vi "Facade.vi"(0 "Data In":T8, 2 "Display State In":T4={"Numeric"=0.0, "Timeline Ref"=refnum, "Waveform Ref"=refnum, "Fill Plots"=FALSE, "Cursor Redraw"=TRUE}, 3 "Container State":T7) -> (6 "Data Out":T8, 7 "Display State Out":T4={"Numeric"=0.0, "Timeline Ref"=refnum, "Waveform Ref"=refnum, "Fill Plots"=FALSE, "Cursor Redraw"=TRUE}, 8 "Action":T3)   [LabVIEW 2017, in "XGrapher.xctl"]
uses:
  XGrapher.xctl
  Data 1.ctl
  Typedefs/Xctrl-Data array.ctl
  Typedefs/Xcrtl-Data format definition.ctl
  Typedefs/Xctl-XY data type definition.ctl
  Typedefs/Xctrl-ROI type enum.ctl
  <vilib>/_xctls/Container State.ctl
  State 1.ctl
  Typedefs/Xctrl-Timeline graph ref.ctl
  Typedefs/Xctrl-Waveform graph ref.ctl
  <vilib>/_xctls/Action.ctl
  Typedefs/Xinformation.ctl
  Typedefs/Xcrtl-Click Operation.ctl
  <vilib>/Utility/miscctls.llb/LVPointTypeDef.ctl
  Globals/gl_X-Grapher refs.vi
  <vilib>/_xctls/XControlSupport.lvlib
panel:
  out "Points in graph":i32 format="%.0f points"
  out "Mouse coordinates info":string="Mouse: X=0, Y=0"
  out "Graph cursor coordinates info":string="Graph cursor: X=0, Y=0"
  out "Xinformation":T1
  out "XY Graph":T13(graph)
  out "Points in timeline":i32 format="%.0f points"
  out "Timeline Graph":T13(graph)
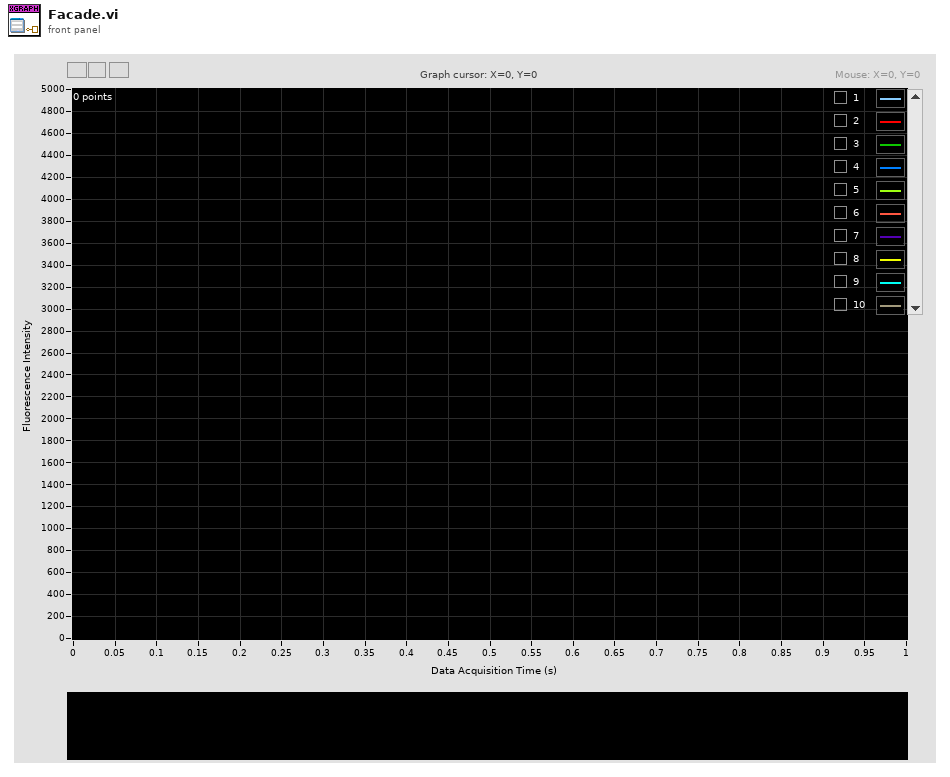
[diagram p1: front panel]
types:
  T1 = typedef "XGrapher.xctl/Xinformation.ctl" = cluster{"Cursor Span":dbl, "Icon":u16, "Mouse Down":bool, "Owning VI":refnum<vi>, "Mouse area":T2, "Dragging":bool, "Drag Offset":dbl, "Original Cursor Pos":cluster{"Left":dbl, "Right":dbl, "Span":dbl}, "Cursor Redraw":bool}
  T2 = typedef "XGrapher.xctl/Xcrtl-Click Operation.ctl" = enum16{"Move", "left cursor", "right cursor", "none"}
  T3 = typedef "XControlSupport.lvlib/Action.ctl" = cluster{"Data Changed?":bool, "State Changed?":bool, "Action Name":string}
  T4 = typedef "XGrapher.xctl/State 1.ctl" = cluster{"Numeric":dbl, "Timeline Ref":T5, "Waveform Ref":T6, "Fill Plots":bool, "Cursor Redraw":bool}
  T5 = typedef "XGrapher.xctl/Xctrl-Timeline graph ref.ctl" = refnum<vi>
  T6 = typedef "XGrapher.xctl/Xctrl-Waveform graph ref.ctl" = refnum<vi>
  T7 = typedef "XControlSupport.lvlib/Container State.ctl" = cluster{"Indicator?":bool, "Run Mode?":bool, " Refnum":refnum<vi>}
  T8 = typedef "XGrapher.xctl/Data 1.ctl" = cluster{"Data & info by ROI index":T9, "Index of selected plot":u16, "Points in each trial":i32, "POI Averaging":bool, "Reset graph X-axis scaling":bool, "Selected point index in MSCN (unity based)":u16}
  T9 = typedef "Xctrl-Data array.ctl" = T10[]
  T10 = typedef "XGrapher.xctl/Xcrtl-Data format definition.ctl" = cluster{"Plot.Plot Name":string, "Data":T11, "Timeline data":T11, "Type":T12, "Points per cycle":u16, "ROI index":u16}
  T11 = typedef "XGrapher.xctl/Xctl-XY data type definition.ctl" = cluster{"X-Axis values":sgl[], "Y-Axis values (s)":sgl[]}
  T12 = typedef "Xctrl-ROI type enum.ctl" = enum16{"POI", "Mini-scan", "Group"}
  T13 = cluster{"X-Axis values":sgl[], "Y-Axis values (s)":sgl[]}[]
  T14 = typedef "LVPointTypeDef.ctl" = cluster{"Horizontal":i16, "Vertical":i16}
  T15 = cluster{"XY Graph":refnum<vi>, "Timeline Graph":refnum<vi>}
  T16 = typedef "XGrapher.xctl/Xctrl-XY Graph data type definition.ctl" = T11[]
  T17 = typedef "LVPoint32TypeDef.ctl" = cluster{"Horizontal":i32, "Vertical":i32}
  T18 = typedef "LVRangeTypeDef.ctl" = cluster{"Minimum":dbl, "Maximum":dbl, "Increment":dbl, "Minor Increment":dbl, "Start":dbl}
  T19 = typedef "lveventtype.ctl" = enum32{"Null", "Timeout", "Annotation Menu Selection", "Annotation Menu Selection?", "App Instance Close", "App Instance Close?", "Autoscale Range Change", "Bookmark Info Change", "Cell Edit", "Cell Edit?", "Cursor Grab", "Cursor Grab?", "Cursor Menu Selection", "Cursor Menu Selection?", "Cursor Move", "Cursor Release", "Data Change", "Direction Change", "Display State Change", "Drag Ended", "Drag Enter", "Drag Leave", "Drag Over", "Drag Source Update", "Drag Starting", "Drag Starting?", "Drop", "Exec State Change", "Key Down", "Key Down?", "Key Repeat", "Key Repeat?", "Key Up", "Listbox Double Click", "Menu Activation?", "Menu Selection (App)", "Menu Selection? (App)", "Menu Selection (User)", "Mouse Down", "Mouse Down?", "Mouse Enter", "Mouse Leave", "Mouse Move", "Mouse Up", "Mouse Wheel", "NI Security User Change (App)", "Pane Size", "Panel Close", "Panel Close?", "Panel Resize", "Plot Attribute Change", "Scale Range Change", "Shortcut Menu Activation?", "Shortcut Menu Selection (App)", "Shortcut Menu Selection? (App)", "Shortcut Menu Selection (User)", "Tree Double Click", "Tree Drag", "Tree Drag?", "Tree Drop", "Tree Drop?", "Tree Item Close", "Tree Item Close?", "Tree Item Open", "Tree Item Open?", "User Event", "Value Change"}
  T20 = cluster{"Left cursor pos.":dbl, "Left cursor pos.":dbl}
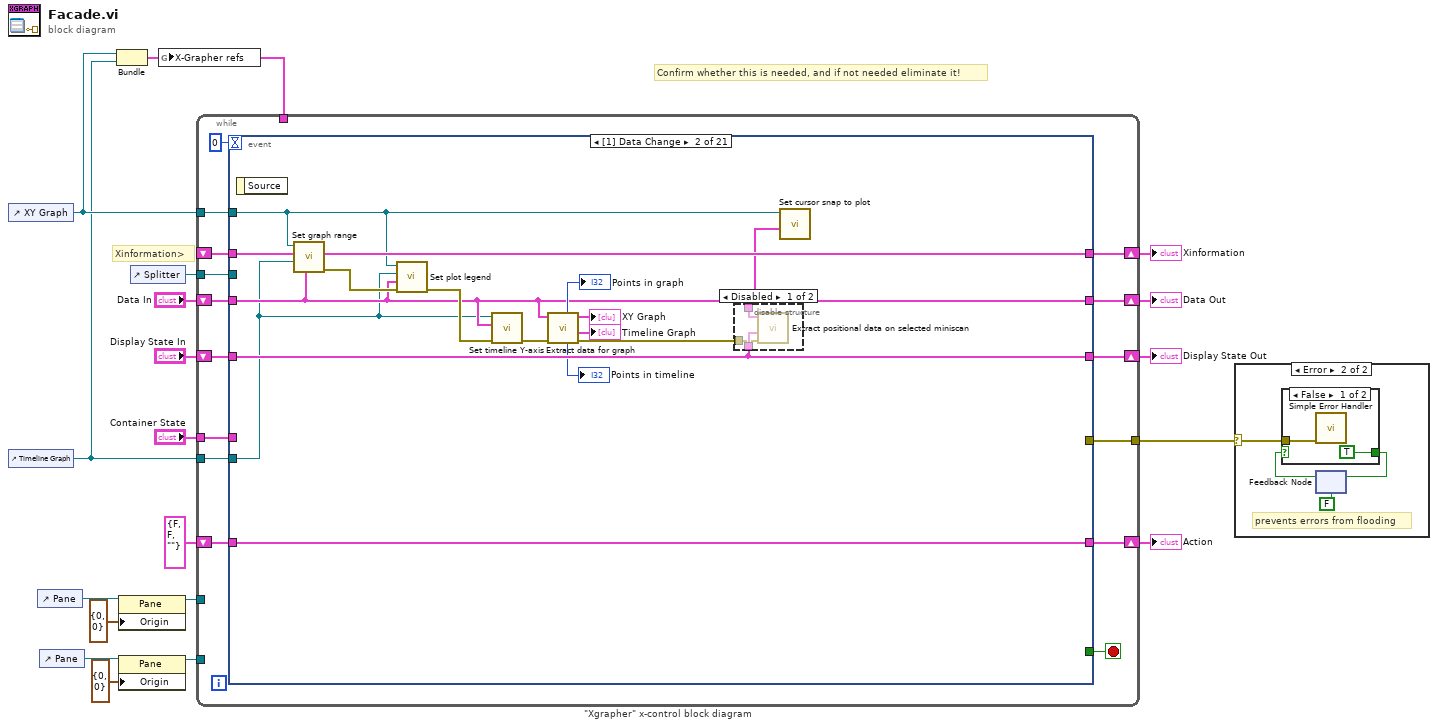
[diagram p0: block diagram]
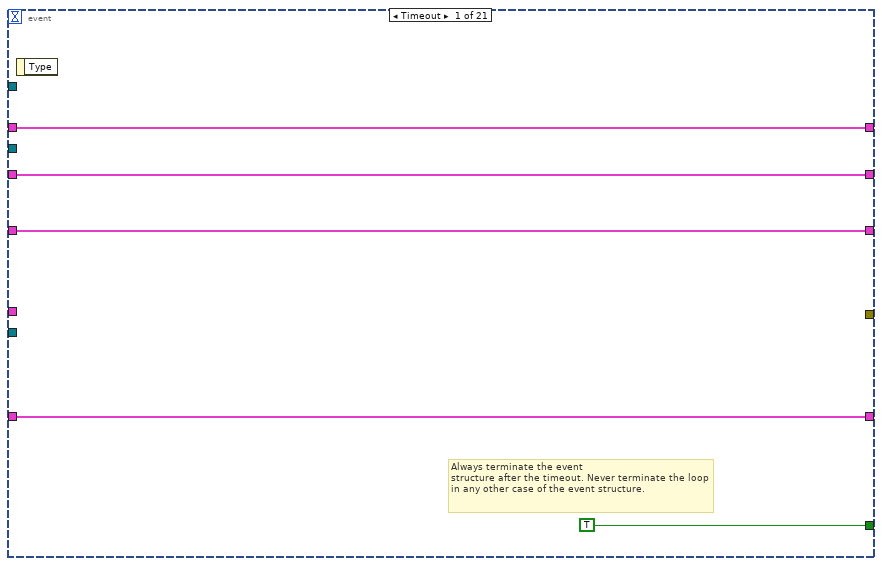
[diagram p4: hidden frame]
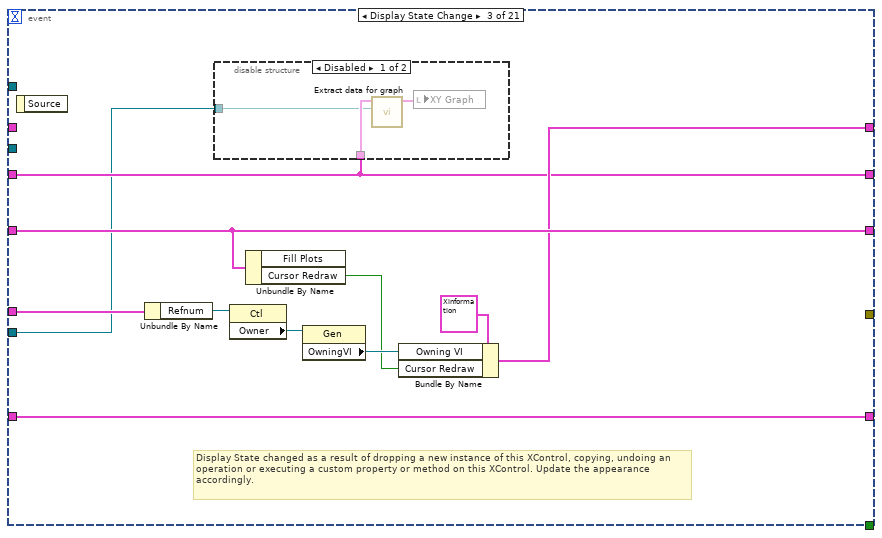
[diagram p6: hidden frame]
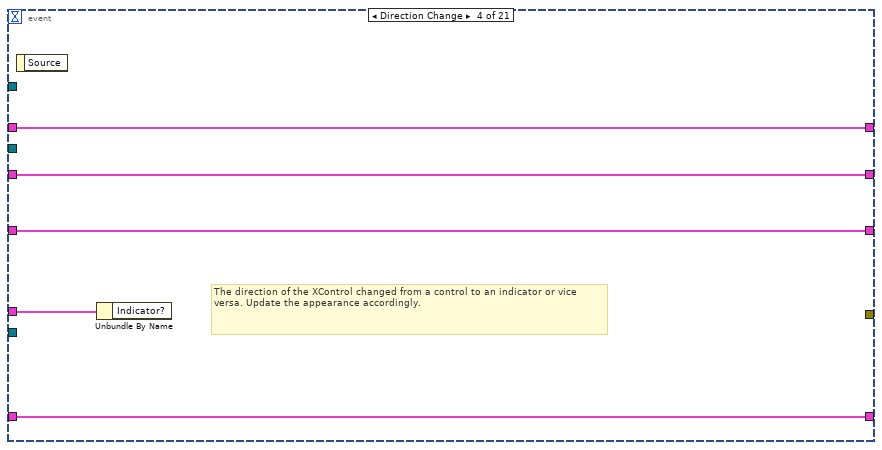
[diagram p8: hidden frame]
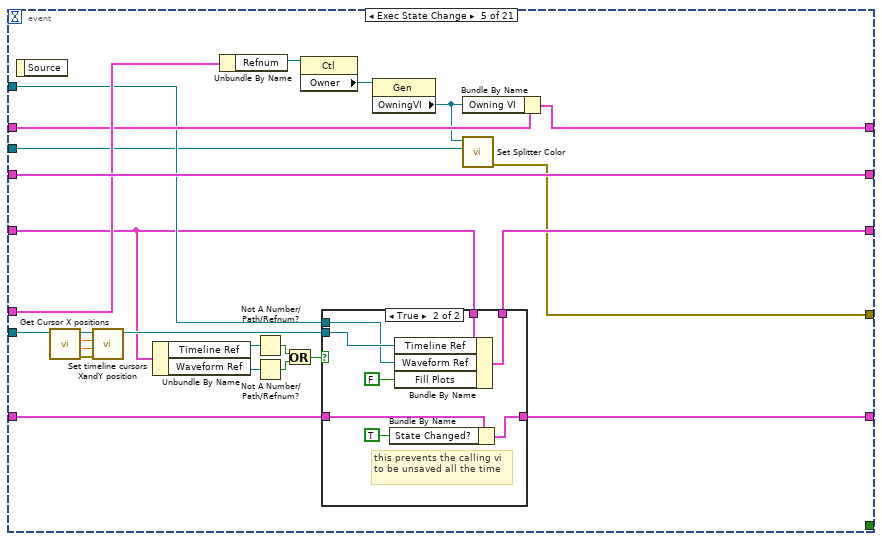
[diagram p9: hidden frame]
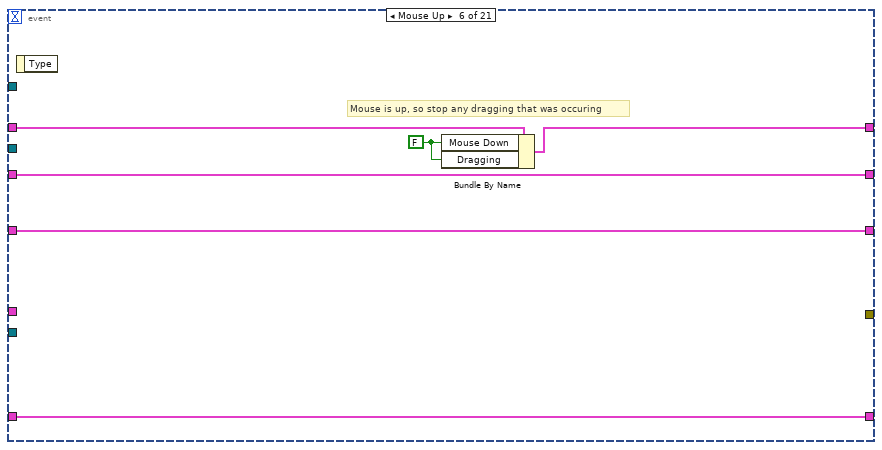
[diagram p11: hidden frame]
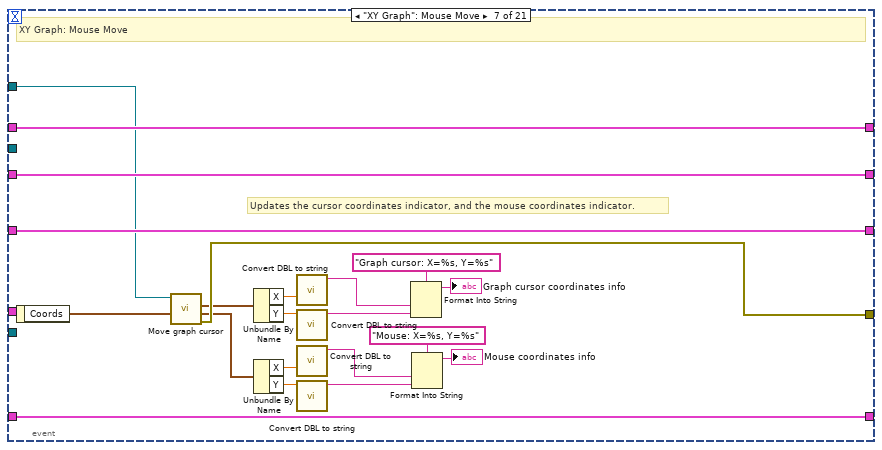
[diagram p12: hidden frame]
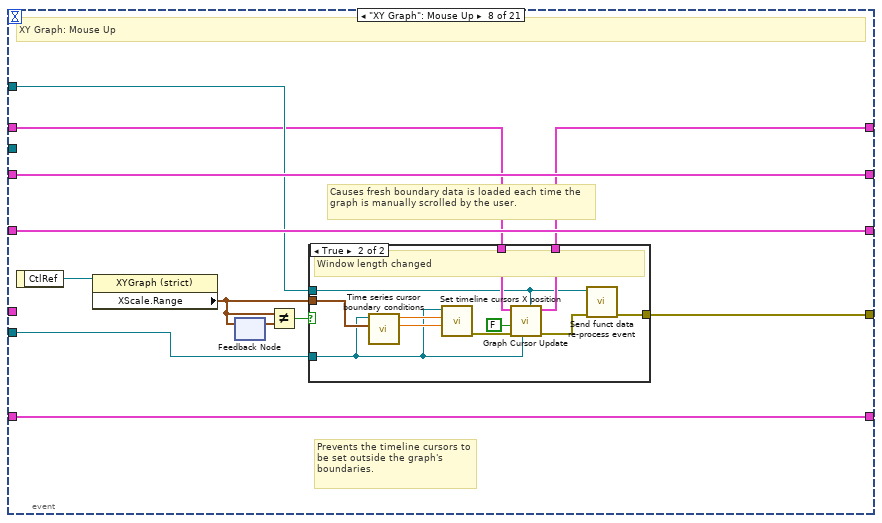
[diagram p13: hidden frame]
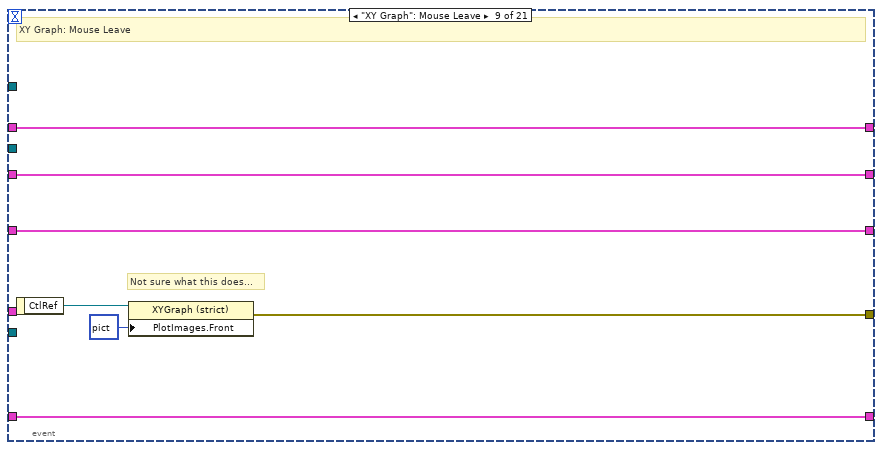
[diagram p15: hidden frame]
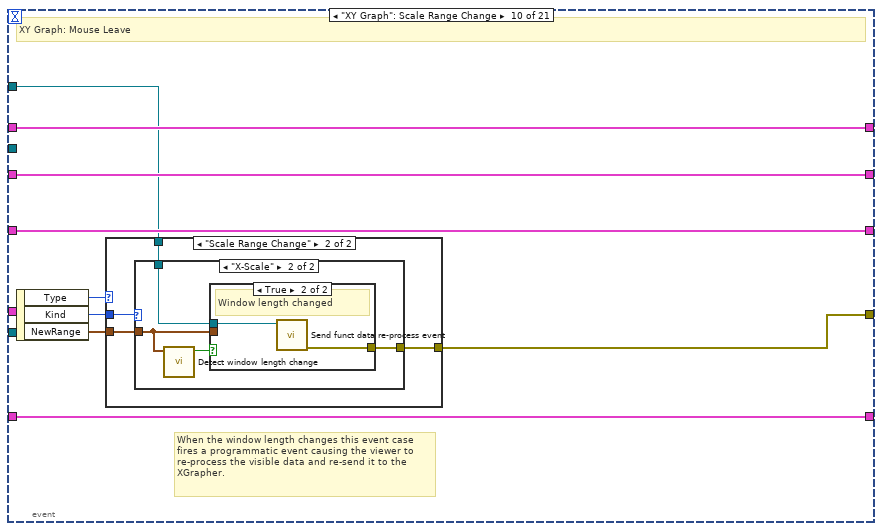
[diagram p16: hidden frame]
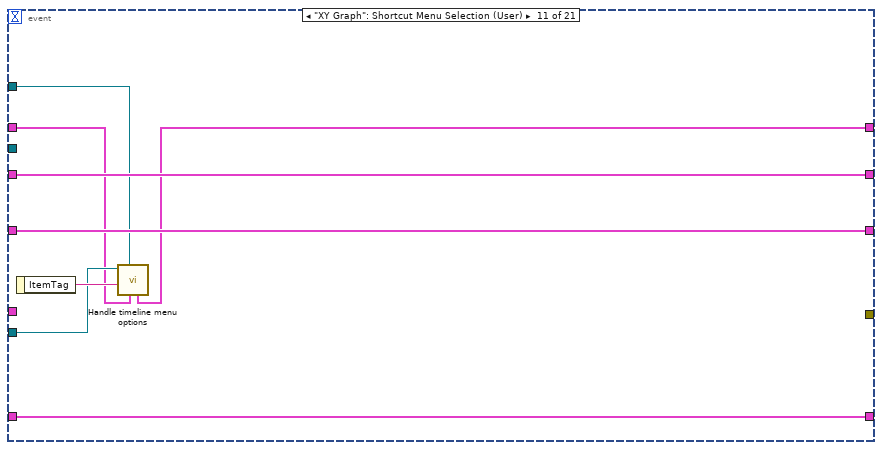
[diagram p20: hidden frame]
diagram:
  # "Confirm whether this is needed, and if not needed eliminate it!"
  # "Xinformation>"
  n1 = control-ref of="XY Graph"() -> (w3:refnum<vi>)
  n2 = control-ref of="Timeline Graph"() -> (w2:refnum<vi>)
  n3 = control-ref of="Pane"() -> (w9:refnum<vi>)
  n4 = control-ref of="Pane"() -> (w7:refnum<vi>)
  n5 = Bundle("XY Graph"=w3, "Timeline Graph"=w2) -> (w1:T15)  [unwired: 1 in]
  n6 = property class="Pane"(reference=w9, "Origin"=T14 {"Horizontal"=0, "Vertical"=0}) -> (reference out=w8:refnum<vi>)  [unwired: 1 in, 1 out]
  n7 = property class="Pane"(reference=w7, "Origin"=T14 {"Horizontal"=0, "Vertical"=0}) -> (reference out=w5:refnum<vi>)  [unwired: 1 in, 1 out]
  n8 = control-ref of="Splitter"() -> (w4:refnum<vi>)
  n9 = global write "gl_X-Grapher refs.vi" "X-Grapher refs"(w1) -> ()
  n10 = while "\"Xgrapher\" x-control block diagram" {
    shift-right: [w33] -> w15
    shift-left: "Display State In" -> [w34]
    tunnel: "Container State" -> [w30]
    shift-right: [w28] -> w19
    shift-left: "Data In" -> [w29]
    shift-right: [w26] -> w17
    shift-left: T3 {"Data Changed?"=FALSE, "State Changed?"=FALSE, "Action Name"=""} ("Action") -> [w27]
    shift-right: [w25] -> w13
    shift-left: _ -> [w24]
    tunnel: [w23] -> w12
    tunnel: w2 -> [w22]
    tunnel: w3 -> [w21]
    tunnel: w8 -> [_]
    tunnel: w5 -> [_]
    tunnel: w4 -> [w20]
    tunnel: w1 -> [_]
    stop <- w32 stop-if-true
    n11 = event shown="[1] Data Change" {
      selector: _ -> [_ _ _ _ _ _ _ _ _ _ _ _ _ _ _ _ _ _ _ _ _]
      dyn-events: _ -> [_ _ _ _ _ _ _ _ _ _ _ _ _ _ _ _ _ _ _ _ _]
      timeout: 0 -> [_ _ _ _ _ _ _ _ _ _ _ _ _ _ _ _ _ _ _ _ _]
      tunnel: w34 -> [w37 w53 w64 w75 w79 w117 w138 w149 w169 w178 w196 w198 w224 w239 w241 w266 w282 w315 w348 w372 w384]
      tunnel: [w37 w53 w64 w75 w94 w117 w138 w149 w169 w178 w196 w198 w224 w239 w241 w266 w282 w314 w348 w372 w384] -> w33
      tunnel: [TRUE _ _ _ _ _ _ _ _ _ _ _ _ _ _ _ _ _ _ _ _] -> w32
      tunnel: w30 -> [_ _ w65 w76 w89 _ _ _ _ _ _ _ _ _ _ _ _ _ _ _ _]
      tunnel: w29 -> [w36 w42 w59 w74 w98 w116 w135 w150 w168 w177 w195 w199 w222 w238 w242 w267 w297 w309 w349 w374 w382]
      tunnel: [w36 w42 w59 w74 w98 w116 w135 w150 w168 w177 w195 w199 w222 w238 w242 w267 w297 w309 w349 w374 w382] -> w28
      tunnel: [w38 w54 w68 w73 w95 w115 w137 w148 w167 w176 w194 w217 w228 w237 w247 w272 w296 w316 w358 w373 w383] -> w26
      tunnel: w27 -> [w38 w54 w68 w73 w96 w115 w137 w148 w167 w176 w194 w217 w228 w237 w247 w272 w296 w316 w358 w373 w383]
      tunnel: [w35 w47 w63 w72 w99 w113 w136 w139 w166 w175 w189 w216 w227 w234 w248 w270 w293 w312 w350 w369 w379] -> w25
      tunnel: w24 -> [w35 w48 _ w72 w88 w114 w136 w140 w166 w175 w190 w216 w220 w235 w243 w271 w294 w299 w355 w370 w379]
      tunnel: [_ _ _ _ w87 _ w134 w143 w163 w174 _ w197 w219 w233 w245 w265 w283 w308 w353 w366 w375] -> w23
      tunnel: w22 -> [_ w40 w58 _ w81 _ _ w142 _ _ w191 w202 _ _ w240 _ _ w302 w351 w367 w376]
      tunnel: w21 -> [_ w41 _ _ w85 _ w132 w144 _ w170 w192 _ w221 _ w244 w264 _ w300 w352 _ _]
      tunnel: w20 -> [_ _ _ _ w77 _ _ _ _ _ _ _ _ _ _ _ _ _ _ _ _]
      event Timeout {
        # "Always terminate the event\nstructure after the timeout. Never terminate the loop in any other case of the event structure."
        n12 = event-data() -> ()  [unwired: 1 in, 1 out]
      }
      event Data Change {
        n13 = event-data() -> ()  [unwired: 1 in, 1 out]
        n14 = call "Set graph range.vi"("Data In"=w42, "Timeline"=w40, "Xinformation Out in"=w48, "XYGraph in"=w41) -> ("error out"=w44:errorcluster, "Xinformation Out out"=w47:T1)  [unwired: 6 in]
        n15 = call "Set plot legend.vi"("error in (no error)"=w44, "Data In"=w42, "Timeline"=w40, "XYGraph in"=w41) -> ("error out"=w43:errorcluster)  [unwired: 6 in, 1 out]
        n16 = call "Set timeline Y-axis.vi"("error in (no error)"=w43, "Data In"=w42, "Timeline Graph in"=w40) -> ("error out"=w49:errorcluster)  [unwired: 7 in, 1 out]
        n17 = call "Extract data for graph.vi"("error in (no error)"=w49, "Data In"=w42) -> ("error out"=w45:errorcluster, "Formatted data for TimeLine graph"=→"Timeline Graph":T16, "Formatted data for main graph"=→"XY Graph":T16, "Number of points in Timeline graph"=→"Points in timeline":i32, "Number of points in main graph"=→"Points in graph":i32)  [unwired: 5 in]
        n18 = disable-structure shown="Disabled" {
          disable-tunnel: w53 -> [w57 _]
          disable-tunnel: w45 -> [w56 _]
          disable-tunnel: w42 -> [w55 _]
          frame Disabled {
            n19 = call "Extract positional data on selected miniscan.vi"("error in (no error)"=w56, "Display State In"=w57, "Data In"=w55) -> ()  [unwired: 7 in, 2 out]
          }
          frame Enabled {
          }
        }
        n20 = call "Set cursor snap to plot.vi"("Data In"=w42, "Waveform Graph in"=w41) -> ()  [unwired: 9 in, 1 out]
      }
      event Display State Change {
        # "Display State changed as a result of dropping a new instance of this XControl, copying, undoing an operation or executing a custom property or method on this XControl. Update the appearance accordingly."
        n21 = event-data() -> ()  [unwired: 1 in, 1 out]
        n22 = Unbundle By Name(w65) -> ("Refnum"=w66:refnum<vi>)
        n23 = disable-structure shown="Disabled" {
          disable-tunnel: w59 -> [w71 _]
          disable-tunnel: w58 -> [w69 _]
          frame Disabled {
            n24 = call "Extract data for graph.vi"(10:w69, "Data In"=w71) -> ("Formatted data for main graph"=w70:T16)  [unwired: 5 in, 4 out]
            n25 = local write "XY Graph"(w70) -> ()
          }
          frame Enabled {
          }
        }
        n26 = property class="Ctl"(reference=w66) -> ("Owner"=w67:refnum<vi>)  [unwired: 1 in, 2 out]
        n27 = Unbundle By Name(w64) -> ("Cursor Redraw"=w60:bool)  [unwired: 1 out]
        n28 = property class="Gen"(reference=w67) -> ("OwningVI"=w62:refnum<vi>)  [unwired: 1 in, 2 out]
        n29 = Bundle By Name(cluster=T1 {"Cursor Span"=0.0, "Icon"=0, "Mouse Down"=FALSE, "Owning VI"=refnum, "Mouse area"=enum."Move", "Dragging"=FALSE, "Drag Offset"=0.0, "Original Cursor Pos"={"Left"=0.0, "Right"=0.0, "Span"=0.0}, "Cursor Redraw"=TRUE} ("Cluster 2"), "Owning VI"=w62, "Cursor Redraw"=w60) -> (w63:T1)
      }
      event Direction Change {
        # "The direction of the XControl changed from a control to an indicator or vice versa. Update the appearance accordingly."
        n30 = event-data() -> ()  [unwired: 1 in, 1 out]
        n31 = Unbundle By Name(w76) -> ()  [unwired: 1 out]
      }
      event Exec State Change {
        n32 = event-data() -> ()  [unwired: 1 in, 1 out]
        n33 = call "Get Cursor X positions.vi"("Timeline Graph"=w81) -> ("error out"=w84:errorcluster, "Right cursor pos."=w83:dbl, "Left cursor pos."=w82:dbl, "Timeline Graph out"=w80:T5)  [unwired: 6 in, 1 out]
        n34 = call "Set timeline cursors XandY position.vi"("error in (no error)"=w84, "Right"=w83, "Left"=w82, "Timeline Graph in"=w80) -> ("Timeline Graph out"=w86:T5)  [unwired: 6 in, 1 out]
        n35 = Unbundle By Name(w79) -> ("Timeline Ref"=w97:T5, "Waveform Ref"=w93:T6)
        n36 = Unbundle By Name(w89) -> ("Refnum"=w100:refnum<vi>)
        n37 = Not A Number/Path/Refnum?(number/path/refnum=w97) -> (NaN/Path/Refnum?=w91:bool)
        n38 = Not A Number/Path/Refnum?(number/path/refnum=w93) -> (NaN/Path/Refnum?=w92:bool)
        n39 = Or(x=w91, y=w92) -> (x .or. y?=w90:bool)
        n40 = property class="Ctl"(reference=w100) -> ("Owner"=w101:refnum<vi>)  [unwired: 1 in, 2 out]
        n41 = case shown="True" w90 {
          tunnel: [w102 w111] -> w94
          tunnel: w96 -> [w103 w110]
          tunnel: [w103 w109] -> w95
          tunnel: w79 -> [w102 w108]
          tunnel: w86 -> [_ w105]
          tunnel: w85 -> [_ w104]
          frame False {
          }
          frame True {
            # "this prevents the calling vi to be unsaved all the time"
            n42 = Bundle By Name(cluster=w110, "State Changed?"=TRUE) -> (w109:T3)
            n43 = Bundle By Name(cluster=w108, "Timeline Ref"=w105, "Waveform Ref"=w104, "Fill Plots"=FALSE) -> (w111:T4)
          }
        }
        n44 = property class="Gen"(reference=w101) -> ("OwningVI"=w78:refnum<vi>)  [unwired: 1 in, 2 out]
        n45 = Bundle By Name(cluster=w88, "Owning VI"=w78) -> (w99:T1)
        n46 = call "Set Splitter Color.vi"("Splitter Refnum"=w77, "OwningVI"=w78) -> ("error out"=w87:errorcluster)  [unwired: 9 in]
      }
      event Mouse Up {
        w112 = FALSE ("Mouse Down")
        # "Mouse is up, so stop any dragging that was occuring"
        n47 = event-data() -> ()  [unwired: 1 in, 1 out]
        n48 = Bundle By Name(cluster=w114, "Mouse Down"=w112, "Dragging"=w112) -> (w113:T1)
      }
      event "XY Graph": Mouse Move {
        # "Updates the cursor coordinates indicator, and the mouse coordinates indicator."
        # "XY Graph: Mouse Move"
        n49 = event-data() -> ("Coords"=w133:T17)  [unwired: 1 in]
        n50 = call "Move graph cursor.vi"("Coords"=w133, "Graph Ref in"=w132) -> ("error out"=w134:errorcluster, "Mouse coordinates"=w120:cluster{"X":dbl, "Y":dbl}, "Graph cursor coordinates"=w125:cluster{"X":dbl, "Y":dbl})  [unwired: 6 in, 1 out]
        n51 = Unbundle By Name(w125) -> ("X"=w124:dbl, "Y"=w123:dbl)
        n52 = Unbundle By Name(w120) -> ("X"=w121:dbl, "Y"=w122:dbl)
        n53 = call "Convert DBL to string.vi"("DBL Value"=w124) -> ("Converted to String"=w130:string)  [unwired: 10 in]
        n54 = call "Convert DBL to string.vi"("DBL Value"=w123) -> ("Converted to String"=w128:string)  [unwired: 10 in]
        n55 = call "Convert DBL to string.vi"("DBL Value"=w121) -> ("Converted to String"=w119:string)  [unwired: 10 in]
        n56 = call "Convert DBL to string.vi"("DBL Value"=w122) -> ("Converted to String"=w118:string)  [unwired: 10 in]
        n57 = Format Into String(format string="Graph cursor: X=%s, Y=%s", w130, w128) -> (resulting string=→"Graph cursor coordinates info":string)  [unwired: 2 in, 1 out]
        n58 = Format Into String(format string="Mouse: X=%s, Y=%s", w119, w118) -> (resulting string=→"Mouse coordinates info":string)  [unwired: 2 in, 1 out]
      }
      event "XY Graph": Mouse Up {
        # "Prevents the timeline cursors to be set outside the graph's boundaries."
        # "Causes fresh boundary data is loaded each time the graph is manually scrolled by the user."
        # "XY Graph: Mouse Up"
        n59 = event-data() -> ("CtlRef"=w147:refnum<vi>)  [unwired: 1 in]
        n60 = property class="XYGraph (strict)"(reference=w147) -> ("XScale.Range"=w141:T18)  [unwired: 1 in, 2 out]
        n61 = feedback-in #1(w141) -> ()
        n62 = feedback #1() -> (w146:T18)  [unwired: 1 in]
        n63 = Not Equal?(x=w141, y=w146) -> (x != y?=w145:bool)
        n64 = case shown="True" w145 {
          tunnel: [_ w162] -> w143
          tunnel: w144 -> [_ w152]
          tunnel: w142 -> [_ w153]
          tunnel: w141 -> [_ w161]
          tunnel: w140 -> [w151 w155]
          tunnel: [w151 w154] -> w139
          frame False {
          }
          frame True {
            # "Window length changed"
            n65 = call "Time series cursor boundary conditions.vi"("XScale.Range"=w161, "Timeline Graph"=w153) -> ("Maximum"=w159:dbl, "Minimum"=w160:dbl)  [unwired: 8 in]
            n66 = call "Set timeline cursors X position.vi"("Right"=w159, "Left"=w160, "Timeline Graph in"=w153) -> ("error out"=w157:errorcluster)  [unwired: 7 in, 1 out]
            n67 = call "Graph Cursor Update.vi"("Waveform Ref in"=w152, "Timeline Ref in"=w153, "error in (no error)"=w157, "Scale graph X-axis (T)"=FALSE, "Xinformation In"=w155) -> ("error out"=w156:errorcluster, "Xinformation Out"=w154:T1)  [unwired: 4 in, 1 out]
            n68 = call "Send funct data re-process event.vi"("error in (no error)"=w156, "Waveform Graph in"=w152) -> ("error out"=w162:errorcluster)  [unwired: 9 in]
          }
        }
      }
      event "XY Graph": Mouse Leave {
        # "Not sure what this does..."
        # "XY Graph: Mouse Leave"
        n69 = event-data() -> ("CtlRef"=w165:refnum<vi>)  [unwired: 1 in]
        n70 = property class="XYGraph (strict)"(reference=w165, "PlotImages.Front"=picture data[5B] ("Plot Images:Front")) -> (error out=w163:errorcluster)  [unwired: 1 in, 1 out]
      }
      event "XY Graph": Scale Range Change {
        # "When the window length changes this event case fires a programmatic event causing the viewer to re-process the visible data and re-send it to the XGrapher."
        # "XY Graph: Mouse Leave"
        n71 = event-data() -> ("Type"=w172:T19, "Kind"=w173:enum16{"X-Scale", "Y-Scale", "Z-Scale"}, "NewRange"=w171:T18)  [unwired: 1 in]
        n72 = case shown="\"Scale Range Change\"" w172 {
          tunnel: [_ w182] -> w174
          tunnel: w171 -> [_ w181]
          tunnel: w173 -> [_ w180]
          tunnel: w170 -> [_ w179]
          frame Default {
          }
          frame "Scale Range Change" {
            n73 = case shown="\"X-Scale\"" w180 {
              tunnel: [_ w186] -> w182
              tunnel: w181 -> [_ w184]
              tunnel: w179 -> [_ w183]
              frame Default {
              }
              frame "X-Scale" {
                n74 = call "Detect window length change.vi"("NewRange"=w184) -> ("Window length changed"=w185:bool)  [unwired: 10 in]
                n75 = case shown="True" w185 {
                  tunnel: [_ w188] -> w186
                  tunnel: w184 -> [_ _]
                  tunnel: w183 -> [_ w187]
                  frame False {
                  }
                  frame True {
                    # "Window length changed"
                    n76 = call "Send funct data re-process event.vi"("Waveform Graph in"=w187) -> ("error out"=w188:errorcluster)  [unwired: 10 in]
                  }
                }
              }
            }
          }
        }
      }
      event "XY Graph": Shortcut Menu Selection (User) {
        n77 = event-data() -> ("ItemTag"=w193:string)  [unwired: 1 in]
        n78 = call "Handle timeline menu options.vi"("Xinformation In"=w190, "Waveform Ref in"=w192, "ItemTag"=w193, "Timeline Ref in"=w191) -> ("Xinformation Out"=w189:T1)  [unwired: 5 in, 2 out]
      }
      event "Timeline Graph": Shortcut Menu Activation? {
        w208 = "Left" ("item name")
        w212 = "Right" ("item name")
        # "when user right clicks, determine if they are about to invert the cursors,\nif so, disable the menu selection"
        n79 = event-data() -> ("MenuRef"=w213:refnum<k9>, "Coords"=w210:T17)  [unwired: 1 in]
        n80 = invoke on="Invoke Node" class="XYGraph (strict)" method="Map Coords To XY"(reference=w202, "Coords"=w210) -> (reference out=w214:refnum<vi>, error out=w203:errorcluster, "XY"=w215:cluster{"X":dbl, "Y":dbl})  [unwired: 5 in, 4 out]
        n81 = Unbundle By Name(w215) -> ("X"=w206:dbl)
        n82 = call "Get Cursor X positions.vi"("error in"=w203, "Timeline Graph"=w214) -> ("error out"=w204:errorcluster, "Right cursor pos."=w201:dbl, "Left cursor pos."=w200:dbl)  [unwired: 5 in, 2 out]
        n83 = Greater?(x=w206, y=w200) -> (0:w211:bool)
        n84 = Less?(x=w206, y=w201) -> (x < y?=w209:bool)
        n85 = Set Menu Item Info(7:w212, 8:w204, 9:w211, 10:w212, 11:w213) -> (0:w205:errorcluster, 3:w207:refnum<k9>)  [unwired: 2 in]
        n86 = Set Menu Item Info(7:w208, 8:w205, 9:w209, 10:w208, 11:w207) -> (0:w197:errorcluster)  [unwired: 2 in, 1 out]
        n87 = event-data() -> ()  [unwired: 2 in, 1 out]
      }
      event "Timeline Graph": Shortcut Menu Selection (User) {
        w226 = FALSE ("Dragging")
        # "Sets the Timeline graph cursor depending on the right-click menu option the user has selected."
        # "after right click menu is closed\ncode still things user has mouse down"
        n88 = event-data() -> ("CtlRef"=w223:refnum<vi>, "ItemTag"=w225:string)  [unwired: 1 in]
        n89 = call "Handle timeline menu options.vi"("Xinformation In"=w220, "Waveform Ref in"=w221, "ItemTag"=w225, "Timeline Ref in"=w223) -> ("error out"=w219:errorcluster, "Xinformation Out"=w218:T1)  [unwired: 5 in, 1 out]
        n90 = Bundle By Name(cluster=w218, "Mouse Down"=w226, "Dragging"=w226) -> (w227:T1)
      }
      event "Timeline Graph": Cursor Grab {
        # "user grabbed a cursor, record original positions\nin case they accidentally invert them"
        n91 = event-data() -> ("CtlRef"=w236:refnum<vi>, "CursRef"=w232:refnum<vi>)  [unwired: 1 in]
        n92 = property class="Curs"(reference=w232, "Cursor Color"=u32 0) -> (error out=w230:errorcluster)  [unwired: 1 in, 1 out]
        n93 = call "Get Cursor X positions.vi"("error in"=w230, "Timeline Graph"=w236) -> ("error out"=w233:errorcluster, "Cursors"=w229:cluster{"Left":dbl, "Right":dbl, "Span":dbl})  [unwired: 5 in, 3 out]
        n94 = Bundle By Name(cluster=w235, "Original Cursor Pos"=w229) -> (w234:T1)
      }
      event "Timeline Graph": Cursor Move {
        n95 = event-data() -> ()  [unwired: 1 in, 1 out]
        n96 = Unbundle By Name(w243) -> ("Cursor Redraw"=w246:bool)
        n97 = case shown="True" w246 {
          tunnel: w243 -> [w249 w254]
          tunnel: [w249 w253] -> w248
          tunnel: w240 -> [_ w252]
          tunnel: [_ w251] -> w245
          tunnel: w244 -> [_ w250]
          frame False {
            # "Graph redraw deferred"
          }
          frame True {
            # "redraw the main graph while the cursors\nare being moved. (may cause performance issues)"
            # "Graph redraw enabled"
            n98 = call "Graph Cursor Update.vi"("Waveform Ref in"=w250, "Timeline Ref in"=w252, "Xinformation In"=w254) -> ("error out"=w251:errorcluster, "Xinformation Out"=w253:T1)  [unwired: 6 in, 1 out]
          }
        }
      }
      event "Timeline Graph": Cursor Release {
        # "change color back to normal"
        # "Get cursor positions"
        # "perform one final screen redraw"
        n99 = event-data() -> ("CursRef"=w269:refnum<vi>, "CtlRef"=w268:refnum<vi>)  [unwired: 1 in]
        n100 = property class="Curs"(reference=w269, "Cursor Color"=u32 9868950) -> (error out=w258:errorcluster)  [unwired: 1 in, 1 out]
        n101 = call "Get Cursor X positions.vi"("Timeline Graph"=w268) -> ("error out"=w262:errorcluster, "Right cursor pos."=w257:dbl, "Left cursor pos."=w256:dbl, "Timeline Graph out"=w255:T5)  [unwired: 6 in, 1 out]
        n102 = Greater?(x=w256, y=w257) -> (0:w263:bool)
        n103 = case "Are cursors inverted?" shown="True" w263 {
          tunnel: [w274 w275] -> w260
          tunnel: w262 -> [w274 w278]
          tunnel: w255 -> [w273 w280]
          tunnel: w271 -> [_ w281]
          tunnel: [w273 w279] -> w261
          tunnel: w258 -> [_ _]
          frame False {
            # "Cursors are not inverted, i.e. valid"
          }
          frame True {
            # "user inverted cursors, so undo that operation"
            # "Cursors are inverted"
            n104 = Unbundle By Name(w281) -> ("Original Cursor Pos.Left"=w277:dbl, "Original Cursor Pos.Right"=w276:dbl)
            n105 = call "Set timeline cursors X position.vi"("error in (no error)"=w278, "Right"=w276, "Left"=w277, "Timeline Graph in"=w280) -> ("error out"=w275:errorcluster, "Timeline Graph out"=w279:T5)  [unwired: 6 in]
          }
        }
        n106 = call "Graph Cursor Update.vi"("Waveform Ref in"=w264, "Timeline Ref in"=w261, "error in (no error)"=w260, "Xinformation In"=w271) -> ("error out"=w265:errorcluster, "Xinformation Out"=w270:T1)  [unwired: 5 in, 1 out]
        n107 = call "Send funct data re-process event.vi"("error in (no error)"=w265, "Waveform Graph in"=w264) -> ()  [unwired: 9 in, 1 out]
      }
      event "Timeline Graph": Mouse Down {
        # "user pressed down on timeline graph, Record offset of click in case they start to drag. Take mouse down xy and subtract left cursor."
        n108 = event-data() -> ("Coords"=w287:T17, "CtlRef"=w292:refnum<vi>)  [unwired: 1 in]
        n109 = invoke on="Timeline Graph" class="XYGraph (strict)" method="Map Coords To XY"("Coords"=w287) -> ("XY"=w291:cluster{"X":dbl, "Y":dbl})  [unwired: 6 in, 6 out]
        n110 = call "Get Cursor X positions.vi"("Timeline Graph"=w292) -> ("error out"=w283:errorcluster, "Left cursor pos."=w285:dbl, "Cursors"=w286:cluster{"Left":dbl, "Right":dbl, "Span":dbl})  [unwired: 6 in, 2 out]
        n111 = Bundle("Left cursor pos."=w285, "Left cursor pos."=w285) -> (w284:T20)  [unwired: 1 in]
        n112 = Unbundle By Name(w286) -> ("Span"=w288:dbl)
        n113 = Subtract(x=w291, y=w284) -> (x-y=w289:cluster{dbl, dbl})
        n114 = Unbundle(w289) -> (w290:dbl)  [unwired: 1 out]
        n115 = Bundle By Name(cluster=w294, "Mouse Down"=TRUE, "Drag Offset"=w290, "Cursor Span"=w288) -> (w293:T1)
      }
      event "Timeline Graph": Mouse Move {
        n116 = event-data() -> ("Coords"=w303:T17, "CtlRef"=w313:refnum<vi>)  [unwired: 1 in]
        n117 = Unbundle By Name(w299) -> ("Dragging"=w310:bool)
        n118 = call "Click Position.vi"("Timeline Ref"=w313, "Click Coords"=w303) -> ("error out"=w307:errorcluster, "Operation"=w306:T2)  [unwired: 8 in]
        n119 = case "Already Dragging?" shown="False" w310 {
          tunnel: [w325 w327] -> w311
          tunnel: w306 -> [w323 _]
          tunnel: w299 -> [w324 w327]
          tunnel: [w323 Xcrtl-Click_Operation."Move" ("Operation")] -> w298
          frame False {
            n120 = Bundle By Name(cluster=w324, "Mouse area"=w323) -> (w325:T1)
          }
          frame True {
          }
        }
        n121 = case shown="\"right cursor\"" w306 {
          tunnel: [w317 u32 0 u32 9868950 w322] -> w305
          tunnel: [w317 u32 9868950 u32 0 w322] -> w304
          frame "Move" {
            w317 = u32 0
          }
          frame "left cursor" {
          }
          frame "right cursor" {
          }
          frame Default {
            w322 = u32 9868950
          }
        }
        n122 = call "Set timeline cursor color.vi"("Color for Cursor 1"=w304, "Color for Cursor 0"=w305, "Timeline Graph in"=w302) -> ("Timeline Graph out"=w301:T5)  [unwired: 8 in]
        n123 = case shown="\"Move\"" w298 {
          tunnel: w315 -> [w336 w341 w347]
          tunnel: [w336 w341 w347] -> w314
          tunnel: w303 -> [w338 _ _]
          tunnel: w311 -> [w334 w340 w346]
          tunnel: [w335 w340 w345] -> w312
          tunnel: [w331 w339 w343] -> w308
          tunnel: w307 -> [w330 w339 w342]
          tunnel: w301 -> [w329 _ _]
          tunnel: w300 -> [w328 _ _]
          frame "Move" {
            # "Mouse is moving inside selected area of timeline graph\nChange mouse icon to 'hand'\nMove Left and Right cursors accordingly"
            n124 = call "Set Mouse Icon.vi"("error in (no error)"=w330, "icon"=u16 11, "Xinformation In"=w334) -> ("error out"=w332:errorcluster, "Xinformation Out"=w333:T1)  [unwired: 7 in]
            n125 = call "Move Selection.vi"("Waveform Graph"=w328, "Timeline"=w329, "error in (no error)"=w332, "Coords"=w338, "Xinformation In"=w333) -> ("error out"=w331:errorcluster, "Xinformation Out"=w335:T1)  [unwired: 5 in]
          }
          frame Default {
            # "regular mouse move\ndo nothing"
          }
          frame "left cursor", "right cursor" {
            # "Don't do anything, let cursor move case handle this"
            n126 = call "Set Mouse Icon.vi"("error in (no error)"=w342, "icon"=u16 0, "Xinformation In"=w346) -> ("error out"=w343:errorcluster, "Xinformation Out"=w345:T1)  [unwired: 7 in]
          }
        }
      }
      event "Timeline Graph": Mouse Up {
        w357 = FALSE
        n127 = event-data() -> ()  [unwired: 1 in, 1 out]
        n128 = Unbundle By Name(w355) -> ("Dragging"=w356:bool)
        n129 = case "Was the user dragging?" shown="True" w356 {
          tunnel: w355 -> [w359 w365]
          tunnel: [w359 w364] -> w354
          tunnel: [_ w362] -> w353
          tunnel: w352 -> [_ w361]
          tunnel: w351 -> [_ w363]
          frame False {
            # "The user was not dragging"
          }
          frame True {
            # "perform one last cursor update\njust in case there was some lag"
            # "The user was dragging"
            n130 = call "Graph Cursor Update.vi"("Waveform Ref in"=w361, "Timeline Ref in"=w363, "Xinformation In"=w365) -> ("error out"=w360:errorcluster, "Xinformation Out"=w364:T1)  [unwired: 6 in, 1 out]
            n131 = call "Send funct data re-process event.vi"("error in (no error)"=w360, "Waveform Graph in"=w361) -> ("error out"=w362:errorcluster)  [unwired: 9 in]
          }
        }
        n132 = Bundle By Name(cluster=w354, "Mouse Down"=w357, "Dragging"=w357) -> (w350:T1)
      }
      event "Timeline Graph": Mouse Leave {
        w368 = u32 9868950
        # "Mouse left timeline control,\nchange mouse icon back to default"
        n133 = event-data() -> ()  [unwired: 1 in, 1 out]
        n134 = call "Set timeline cursor color.vi"("Color for Cursor 1"=w368, "Color for Cursor 0"=w368, "Timeline Graph in"=w367) -> ()  [unwired: 8 in, 1 out]
        n135 = call "Set Mouse Icon.vi"("icon"=u16 0, "Xinformation In"=w370) -> ("error out"=w366:errorcluster, "Xinformation Out"=w369:T1)  [unwired: 8 in]
      }
      event "Timeline Graph": Scale Range Change {
        # "User inverted cursors, so undo that operation"
        # "the user accidentally changed the range of the timeline,\nchange it back to the original setting"
        n136 = event-data() -> ()  [unwired: 1 in, 1 out]
        n137 = property on="Timeline Graph" class="XYGraph (strict)"("XScale.ScaleFit"=u8 1 ("X Scale.Scale Fit")) -> (error out=w377:errorcluster)  [unwired: 2 in, 1 out]
        n138 = Unbundle By Name(w379) -> ("Original Cursor Pos.Left"=w381:dbl, "Original Cursor Pos.Right"=w380:dbl)
        n139 = call "Set timeline cursors X position.vi"("error in (no error)"=w377, "Right"=w380, "Left"=w381, "Timeline Graph in"=w376) -> ("error out"=w375:errorcluster)  [unwired: 6 in, 1 out]
      }
    }
  }
  "Display State Out" <- w15
  "Data Out" <- w19
  "Action" <- w17
  "Xinformation" <- w13
  n140 = case shown="Error" w12 {
    selector: w12 -> [_ w388]
    frame No Error {
    }
    frame Error {
      # "prevents errors from flooding"
      n141 = feedback #2(FALSE) -> (w386:bool)
      n142 = case shown="False" w386 {
        selector: w386 -> [_ w391]
        tunnel: w388 -> [w390 _]
        tunnel: [TRUE w391] -> w387
        frame False {
          n143 = call <vilib>:"Simple Error Handler.vi"("error in (no error)"=w390) -> ()  [unwired: 4 in, 5 out]
        }
        frame True {
        }
      }
      n144 = feedback-in #2(w387) -> ()
    }
  }
